vi "Get Relative Image Times.vi"(7 "size":u32, 8 "error in (no error)":errorcluster, 9 "arr":cluster{}, 10 "last":u32, 11 "first":u32) -> (0 "error out":errorcluster, 1 "arr out":cluster{}, 3 "function return":u32)   [LabVIEW 2014, in "atmcd32d.lvlib"]
doc: "unsigned int WINAPI GetRelativeImageTimes(unsigned int first, unsigned int last, at_u64 * arr, unsigned int size);"
uses:
  atmcd32d.lvlib
  atmcd32d.dll
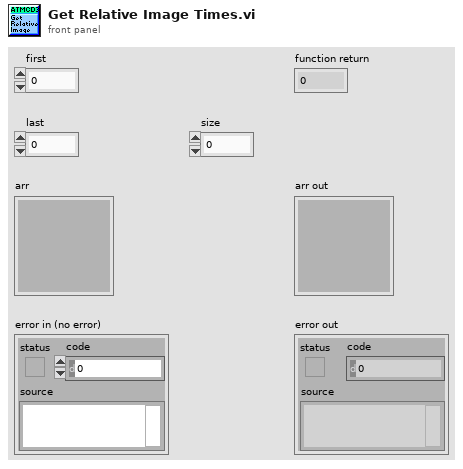
[diagram p1: front panel]
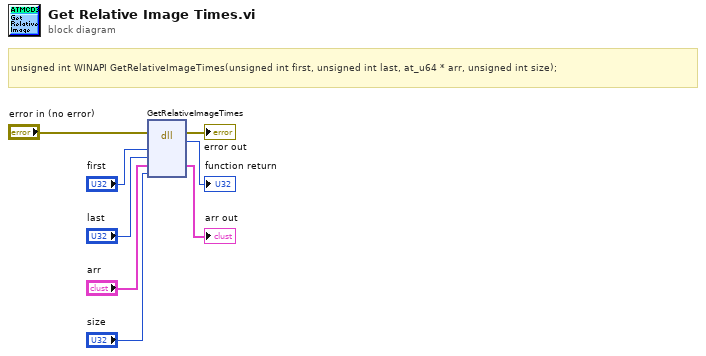
[diagram p0: block diagram]
diagram:
  # "unsigned int WINAPI GetRelativeImageTimes(unsigned int first, unsigned int last, at_u64 * arr, unsigned int size);"
  n1 = dll-call lib="C:/Users/Bakir/Documents/Lambda2-Testing/lib/Andorlib/atmcd32d.*" fn="GetRelativeImageTimes"(error in="error in (no error)", "first"="first", "last"="last", "arr"="arr", "size"="size") -> (error out=→"error out":errorcluster, →"function return":u32, "arr"=→"arr out":cluster{})  [unwired: 5 in, 1 out]
